vi "GetImageFromFileIcon.vi"(7 "Origin":T1, 8 "error in (no error)":errorcluster, 9 "AddFrame":bool, 10 "Bounds":T3, 11 "path to JPEG file":path) -> (0 "error out":errorcluster, 2 "Image Data":T2, 3 "2D Picture Out":picture)   [LabVIEW 2015]
uses:
  <vilib>/Utility/miscctls.llb/LVBoundsTypeDef.ctl
  <vilib>/picture/picture.llb/imagedata.ctl
  <vilib>/Utility/miscctls.llb/LVPoint32TypeDef.ctl
  21_Image/Picture_Class/Picture_Class.lvclass
panel:
  out "2D Picture":picture
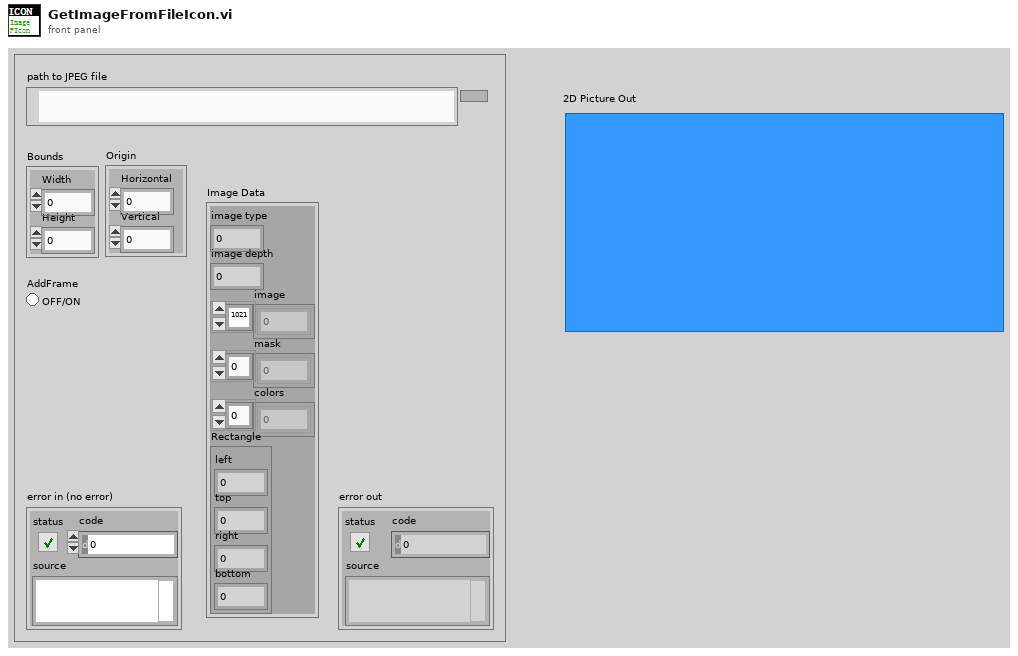
[diagram p1: front panel]
types:
  T1 = typedef "LVPoint32TypeDef.ctl" = cluster{"Horizontal":i32, "Vertical":i32}
  T2 = typedef "imagedata.ctl" = cluster{"image type":i32, "image depth":i32, "image":u8[], "mask":u8[], "colors":u32[], "Rectangle":cluster{"left":i16, "top":i16, "right":i16, "bottom":i16}}
  T3 = typedef "LVBoundsTypeDef.ctl" = cluster{"Width":u32, "Height":u32}
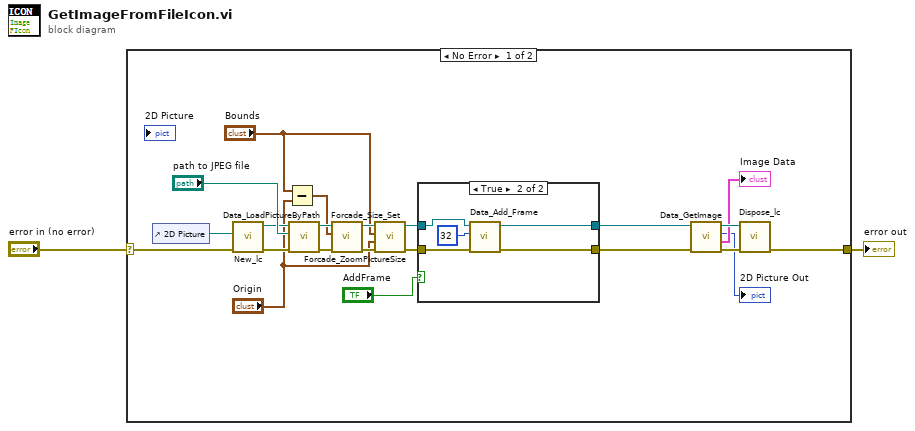
[diagram p0: block diagram]
diagram:
  n1 = case shown="No Error" "error in (no error)" {
    selector: "error in (no error)" -> [w15 w32]
    tunnel: [w16 w32] -> w1
    frame No Error {
      n2 = control-ref of="2D Picture"() -> (w24:refnum<vi>)
      n3 = call "New_lc.vi"("error in (no error)"=w15, "PictureRef"=w24) -> ("error out"=w23:errorcluster, "Picture_Class 输出"=w21:refnum<class "Picture_Class.lvclass">)  [unwired: 8 in]
      n4 = Subtract(x="Bounds", y="Origin") -> (x-y=w9:T3)
      n5 = call "Data_LoadPictureByPath.vi"("error in (no error)"=w23, "Image Path"="path to JPEG file", "Picture_Class 输入"=w21) -> ("error out"=w14:errorcluster, "Picture_Class 输出"=w12:refnum<class "Picture_Class.lvclass">)  [unwired: 7 in]
      n6 = call "Forcade_Size_Set.vi"("error in (no error)"=w14, "Draw Area Size"=w9, "Picture_Class 输入"=w12) -> ("error out"=w13:errorcluster, "Picture_Class 输出"=w11:refnum<class "Picture_Class.lvclass">)  [unwired: 7 in]
      n7 = call "Forcade_ZoomPictureSize.vi"("error in (no error)"=w13, "Origin"="Origin", "Bounds"="Bounds", "Picture_Class 输入"=w11) -> ("error out"=w20:errorcluster, "Picture_Class 输出"=w19:refnum<class "Picture_Class.lvclass">)  [unwired: 4 in, 2 out]
      n8 = case shown="True" "AddFrame" {
        tunnel: w20 -> [w26 w31]
        tunnel: w19 -> [w25 w30]
        tunnel: [w26 w29] -> w7
        tunnel: [w25 w28] -> w17
        frame False {
        }
        frame True {
          n9 = call "Data_Add_Frame.vi"("error in (no error)"=w31, "Width"=i16 32, "Picture_Class 输入"=w30) -> ("error out"=w29:errorcluster, "Picture_Class 输出"=w28:refnum<class "Picture_Class.lvclass">)  [unwired: 7 in]
        }
      }
      n10 = call "Data_GetImage.vi"("error in (no error)"=w7, "Picture_Class 输入"=w17) -> ("error out"=w6:errorcluster, "image data"=→"Image Data":T2, "Picture Out"=→"2D Picture Out":picture, "Picture_Class 输出"=w8:refnum<class "Picture_Class.lvclass">)  [unwired: 6 in]
      n11 = call "Dispose_lc.vi"("error in (no error)"=w6, "Picture_Class 输入"=w8) -> ("error out"=w16:errorcluster)  [unwired: 8 in, 1 out]
    }
    frame Error {
    }
  }
  "error out" <- w1
